vi "xGeneral Cluster to XML.vi"(1 "General Cluster":cluster{"Location":i16} {"Location" items=["Purdue", "NIKHEF", "Zurich", "???"]}, 2 "Input String":string) -> (0 "Output String":string)   [LabVIEW 2012]
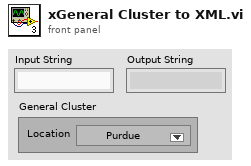
[diagram p1: front panel]
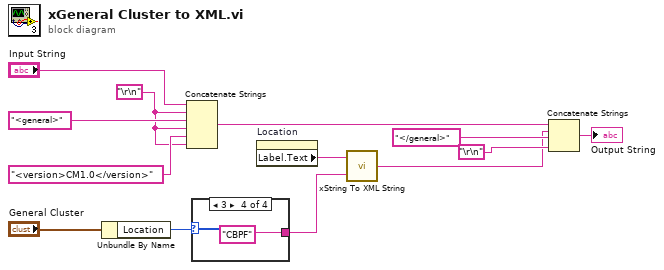
[diagram p0: block diagram]
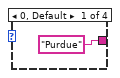
[diagram p2: hidden frame]
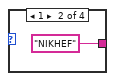
[diagram p3: hidden frame]
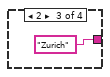
[diagram p4: hidden frame]
diagram:
  w5 = "\r\n"
  n1 = Unbundle By Name("General Cluster") -> ("Location"=w1:i16)
  n2 = Concatenate Strings("Input String", w5, "<general>" ("string"), w5, "<version>CM1.0</version>" ("string"), w5) -> (w10:string)
  n3 = case shown="3" w1 {
    tunnel: ["Purdue" "NIKHEF" "Zurich" "CBPF"] -> w7
    frame 0, Default {
    }
    frame 1 {
    }
    frame 2 {
    }
    frame 3 {
    }
  }
  n4 = property on="Location" class="Ring (strict)"() -> ("Label.Text"=w6:string)  [unwired: 2 in, 2 out]
  n5 = call "xString To XML String.vi"("String to write"=w7, "XML Tag"=w6) -> ("xml string"=w11:string)
  n6 = Concatenate Strings(w10, w11, "</general>" ("string"), "\r\n") -> (→"Output String":string)
